vi "Read RequestedFields.vi"(8 "error in (no error)":errorcluster, 11 "DynamicParameters in":refnum<class "DynamicParameters.lvclass">) -> (0 "error out":errorcluster, 2 "RequestedFields":string[](array[string]), 3 "DynamicParameters out":refnum<class "DynamicParameters.lvclass">)   [LabVIEW 2020, in "ORM.lvlib" / "DynamicParameters.lvclass"]
uses:
  DynamicParameters.lvclass
  DynamicParameters.lvclass/DynamicParameters.ctl
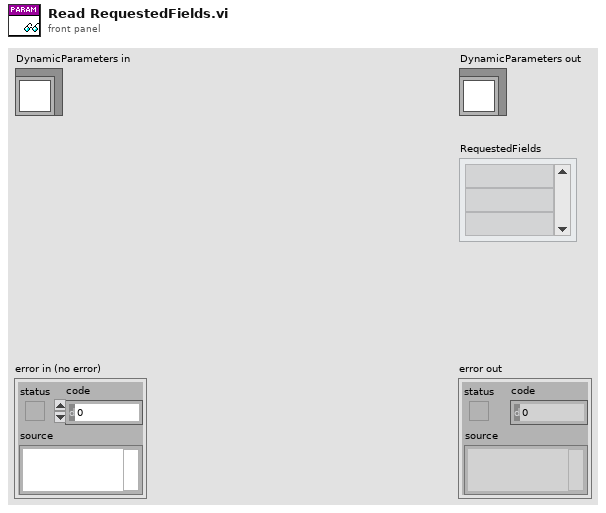
[diagram p1: front panel]
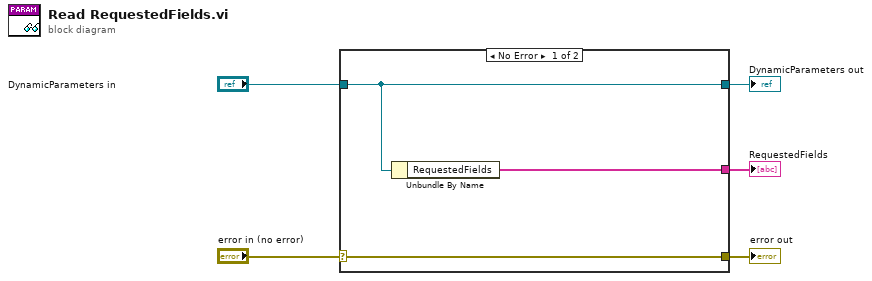
[diagram p0: block diagram]
diagram:
  n1 = case shown="No Error" "error in (no error)" {
    selector: "error in (no error)" -> [w8 w9]
    tunnel: [w8 w9] -> w4
    tunnel: [w7 w10] -> w2
    tunnel: "DynamicParameters in" -> [w7 w10]
    tunnel: [w6 _] -> w1
    frame No Error {
      n2 = Unbundle By Name(w7) -> ("RequestedFields"=w6:string[])
    }
    frame Error {
    }
  }
  "error out" <- w4
  "DynamicParameters out" <- w2
  "RequestedFields" <- w1
